vi "fpga_Lockout Control.vi"(0 "force to lockout state? (F)":bool, 2 "release from lockout? (F)":bool, 5 "reclosing setting":T1={"number of reclosing attempts"=1, "dead times [ms]"=[0, 0, 0, 0, 0, 0, 0], "close pulse duration [ms]"=0, "reclaim time [ms]"=0, "enable synchronism check? (F)"=FALSE, "enable lockout reset? (F)"=FALSE, "lockout reset time [ms]"=0} {"number of reclosing attempts" items=["1"=1, "2"=2, "3"=3, "4"=4, "5"=5, "6"=6, "7"=7]}, 9 "sequence timer active? (F)":bool, 11 "shot count":u8) -> (4 "released from lockout?":bool, 8 "lockout?":bool, 15 "block output during lockout?":bool)   [LabVIEW 2012, in "NI_EP_Protection_FPGA.lvlib"]
uses:
  <vilib>/addons/Electrical Power/Protection/NI_EP_Protection_FPGA.lvlib
  <vilib>/addons/Electrical Power/Protection/Reclosing Logic/subVIs/fpga_Recloser Logic Setting.ctl
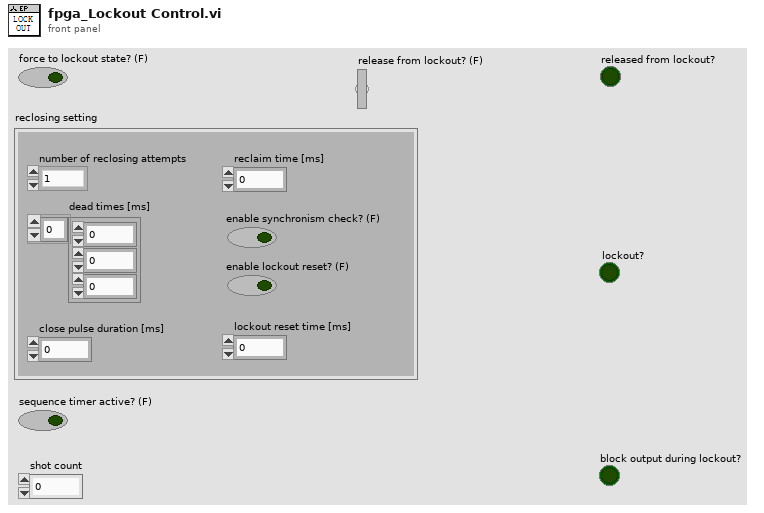
[diagram p1: front panel]
types:
  T1 = typedef "NI_EP_Protection_FPGA.lvlib/fpga_Recloser Logic Setting.ctl" = cluster{"number of reclosing attempts":u8, "dead times [ms]":u32[], "close pulse duration [ms]":u32, "reclaim time [ms]":u32, "enable synchronism check? (F)":bool, "enable lockout reset? (F)":bool, "lockout reset time [ms]":u32}
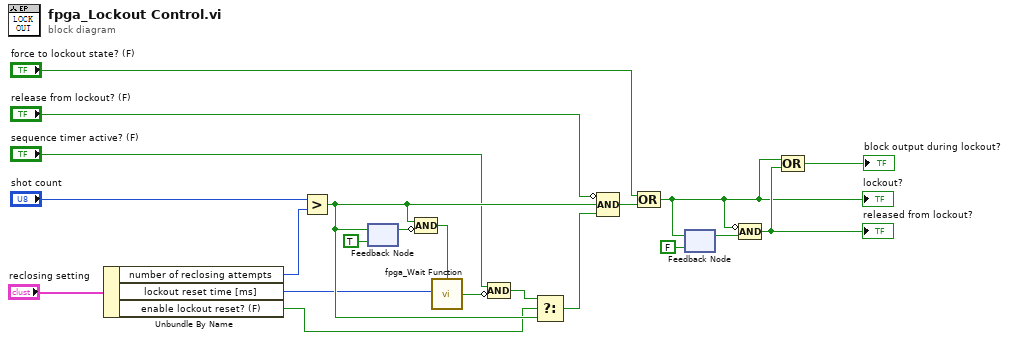
[diagram p0: block diagram]
diagram:
  n1 = Unbundle By Name("reclosing setting") -> ("number of reclosing attempts"=w7:u8, "lockout reset time [ms]"=w8:u32, "enable lockout reset? (F)"=w9:bool)
  n2 = Greater?(x="shot count", y=w7) -> (0:w12:bool)
  n3 = feedback #1(TRUE) -> (w16:bool)
  n4 = feedback-in #1(w12) -> ()
  n5 = Compound Arithmetic op=AND(w12, invert w16) -> (w14:bool)
  n6 = call <vilib>:"fpga_Wait Function.vi"("start? (F)"=w14, "timeout (ms)"=w8) -> ("timeout?"=w6:bool)  [unwired: 13 in]
  n7 = Compound Arithmetic op=AND("sequence timer active? (F)", invert w6) -> (w18:bool)
  n8 = Select(t=w18, s=w9, f=w12) -> (s? t:f=w13:bool)
  n9 = Compound Arithmetic op=AND(invert "release from lockout? (F)", w12, w13) -> (w11:bool)
  n10 = Compound Arithmetic op=OR("force to lockout state? (F)", w11) -> (w4:bool)
  "lockout?" <- w4
  n11 = feedback #2(FALSE) -> (w19:bool)
  n12 = feedback-in #2(w4) -> ()
  n13 = Compound Arithmetic op=AND(invert w4, w19) -> (w5:bool)
  "released from lockout?" <- w5
  n14 = Compound Arithmetic op=OR(w4, w5) -> (→"block output during lockout?":bool)
